vi "FPGA Reference - Get.vi"(8 "error in":errorcluster) -> (0 "error out":errorcluster, 3 "FPGA Reference Out":T1)   [LabVIEW 2024, in "FPGA Interface.lvlib"]
uses:
  FPGA Interface.lvlib
  Type Definitions/ECU FPGA Reference.ctl
  FPGA Ref Action.ctl
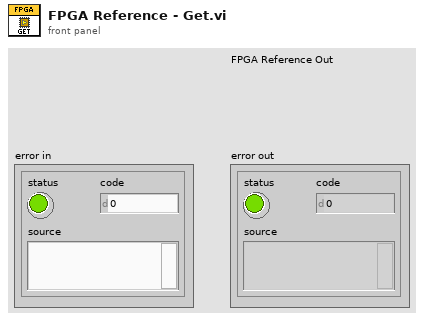
[diagram p1: front panel]
types:
  T1 = typedef "ECU FPGA Reference.ctl" = refnum<k20>
  T2 = typedef "FPGA Interface.lvlib/FPGA Ref Action.ctl" = enum16{"Open Ref", "Get Ref", "Close Ref"}
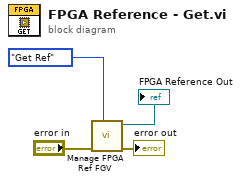
[diagram p0: block diagram]
diagram:
  n1 = call "Manage FPGA Ref FGV.vi"("FPGA Action"=FPGA_Ref_Action."Get Ref", "error in"="error in") -> ("error out"=→"error out":errorcluster, "FPGA Reference Out"=→"FPGA Reference Out":T1)  [unwired: 8 in]
